vi "Initialize UI.vi"(0 "Room Service Monitor UI in":refnum<class "Room Service Monitor UI.lvclass">, 11 "error in (no error)":errorcluster) -> (4 "Room Service Monitor UI out":refnum<class "Room Service Monitor UI.lvclass">, 15 "error out":errorcluster)   [LabVIEW 2023, in "Room Service Monitor UI.lvlib" / "Room Service Monitor UI.lvclass"]
uses:
  Room Service Monitor UI.lvclass
  Room Service Monitor UI.lvclass/Room Service Monitor UI.ctl
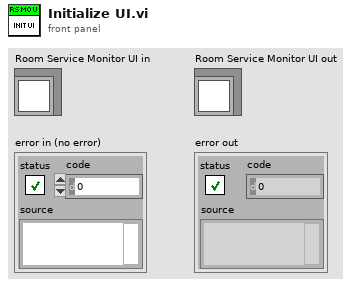
[diagram p1: front panel]
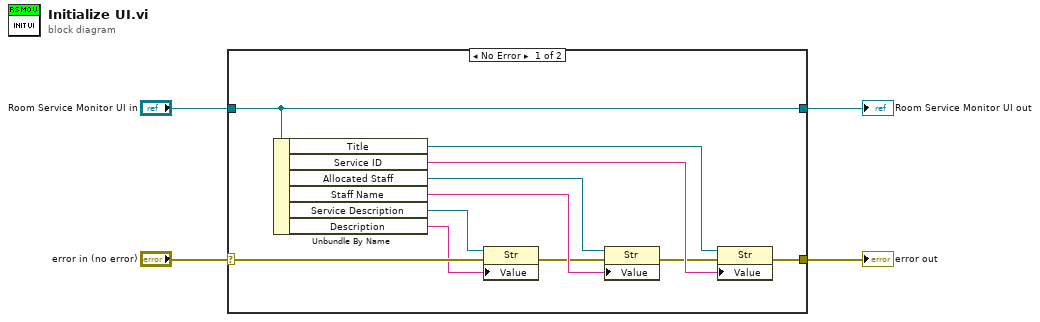
[diagram p0: block diagram]
diagram:
  n1 = case shown="No Error" "error in (no error)" {
    selector: "error in (no error)" -> [w15 w17]
    tunnel: [w14 w17] -> w3
    tunnel: [w13 w16] -> w1
    tunnel: "Room Service Monitor UI in" -> [w13 w16]
    frame No Error {
      n2 = Unbundle By Name(w13) -> ("Title"=w12:refnum<vi>, "Service ID"=w11:string, "Allocated Staff"=w9:refnum<vi>, "Staff Name"=w8:string, "Service Description"=w6:refnum<vi>, "Description"=w5:string)
      n3 = property class="Str"(reference=w6, error in=w15, "Value"=w5) -> (error out=w7:errorcluster)  [unwired: 1 out]
      n4 = property class="Str"(reference=w9, error in=w7, "Value"=w8) -> (error out=w10:errorcluster)  [unwired: 1 out]
      n5 = property class="Str"(reference=w12, error in=w10, "Value"=w11) -> (error out=w14:errorcluster)  [unwired: 1 out]
    }
    frame Error {
    }
  }
  "error out" <- w3
  "Room Service Monitor UI out" <- w1
